vi "String2PieceColor.vi"(1 "String":string) -> (0 "Piece Color":T1)   [LabVIEW 2020]
doc: "From an upper or lowercase string, returns the piece color"
uses:
  Pieces/typedefs/pieceColor.ctl
  Pieces/Piece.lvclass
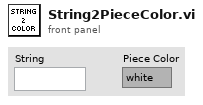
[diagram p1: front panel]
types:
  T1 = typedef "Piece.lvclass/pieceColor.ctl" = enum16{"white", "black"}
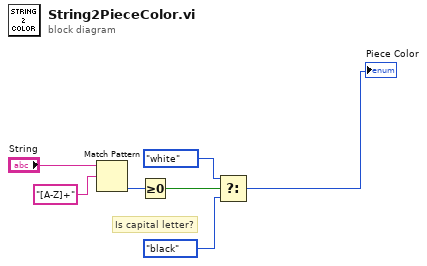
[diagram p0: block diagram]
diagram:
  # "Is capital letter?"
  n1 = Match Pattern(string="String", regular expression="[A-Z]+") -> (offset past match=w2:i32)  [unwired: 1 in, 3 out]
  n2 = Greater Or Equal To 0?(x=w2) -> (x >= 0?=w3:bool)
  n3 = Select(t=pieceColor."white" ("pieceColor"), s=w3, f=pieceColor."black") -> (s? t:f=→"Piece Color":T1)
